vi "add_line_enface_IMAQv2.vi"(6 "Output Line":i32, 7 "Temp Image":T1, 8 "error in (no error)":errorcluster, 9 "Input Line":dbl=74.0, 10 "Raw Image":T1, 11 "En Face Image":T1) -> (0 "error out":errorcluster, 3 "En Face Image Out":T1)   [LabVIEW 2016]
uses:
  <vilib>/vision/Image Controls.llb/IMAQ Image.ctl
  <vilib>/vision/NI_Vision_Development_Module.lvlib
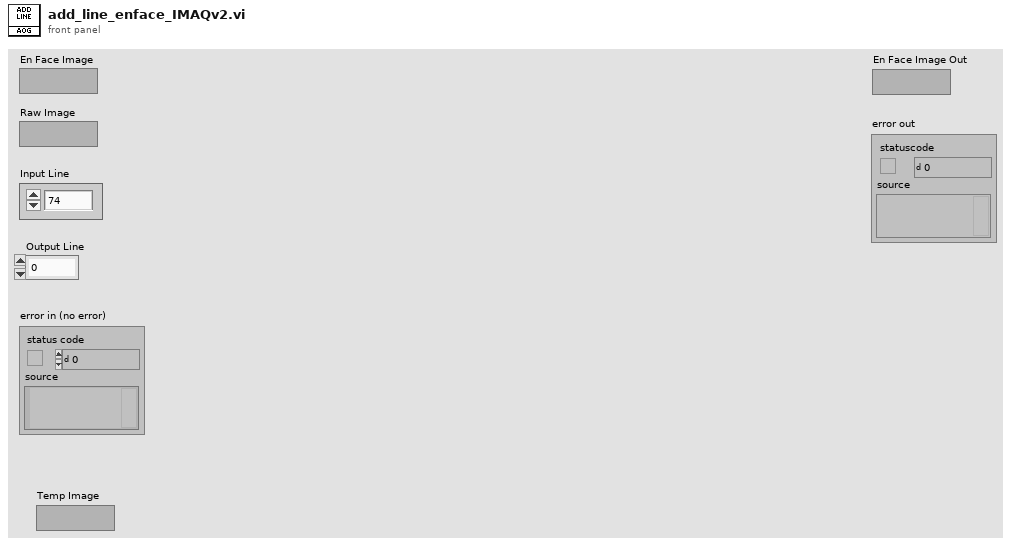
[diagram p1: front panel]
types:
  T1 = typedef "IMAQ Image.ctl" = refnum<image>
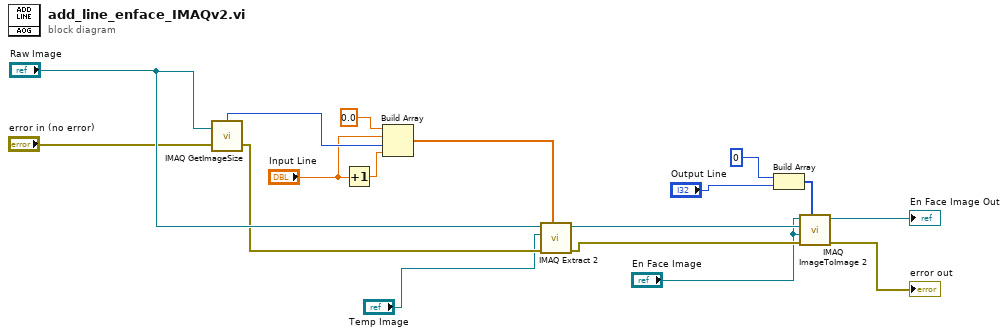
[diagram p0: block diagram]
diagram:
  n1 = call "IMAQ GetImageSize"("Image"="Raw Image", "error in (no error)"="error in (no error)") -> ("X Resolution"=w5:i32, "error out"=w6:errorcluster)  [unwired: 2 in, 1 out]
  n2 = Increment(x="Input Line") -> (x+1=w3:dbl)
  n3 = Build Array(0.0 ("element"), "Input Line", w5, w3) -> (w16:dbl[])
  n4 = call "IMAQ Extract 2"("Optional Rectangle"=w16, "error in (no error)"=w6, "Image Dst"="Temp Image", "Image Src"="Raw Image") -> ("error out"=w7:errorcluster, "Image Dst Out"=w15:T1)  [unwired: 6 in]
  n5 = Build Array(0 ("element"), "Output Line") -> (w11:i32[])
  n6 = call "IMAQ ImageToImage 2"("Offset Left/Top"=w11, "error in (no error)"=w7, "Image Dst"="En Face Image", "Image Src (Small)"=w15, "Image Src (Large)"="En Face Image") -> ("error out"=→"error out":errorcluster, "Image Dst Out"=→"En Face Image Out":T1)  [unwired: 5 in]
